vi "Elapsed_time.vi"() -> ()   [LabVIEW 2020]
panel:
  in  "Numeric":dbl
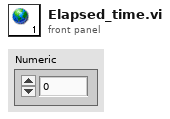
[diagram p1: front panel]
diagram:
